vi "Mutate.vi"() -> ()   [LabVIEW 2014, in "VeriStand Steps Version Mutation.lvlib"]
uses:
  VeriStand Steps Version Mutation.lvlib
  Types/Version Build Information.ctl
  Types/Project Paths Cluster.ctl
  Types/dotNET Config File Paths Cluster.ctl
  <vilib>/Wiresmith Technology/LabVIEW CLI/CLI Class/CLI.lvclass
panel:
  out "error out":errorcluster
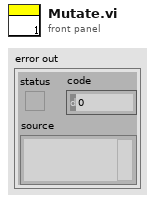
[diagram p1: front panel]
types:
  T1 = typedef "VeriStand Steps Version Mutation.lvlib/Version Build Information.ctl" = cluster{"VeriStand Version":string, "TestStand Version":string, "New VS Assembly Version":string, "New TS Assembly Version":string, "VeriStand Steps Version String":string, "Project Paths":T2, "New TS Interop Assembly Version":string, "New TS Utility Assembly Version":string, "New VS Assembly Version (GAC)":string, "dotNET .config File Paths":T3}
  T2 = typedef "VeriStand Steps Version Mutation.lvlib/Project Paths Cluster.ctl" = cluster{"MiscHelperVIs Project Path":string, "RTSequenceVIs Project Path":string, "Set Channels Project Path":string, "TS VS Logger Project Path":string, "VeriStand.exe Install Path":string, "NI_VeristandTypes.ini File Path":string, "Workspace Path":string, "VeristandSteps.csproj File Path":string, "Silent Veristand Project Path":string}
  T3 = typedef "VeriStand Steps Version Mutation.lvlib/dotNET Config File Paths Cluster.ctl" = cluster{"MiscHelperVIs Project .config File Path":path, "RT Sequence VIs Project .config File Path":path, "Set Channels Project .config File Path":path, "TS VS Logger Project .config File Path":path, "Silent Veristand Project .config File Path":path}
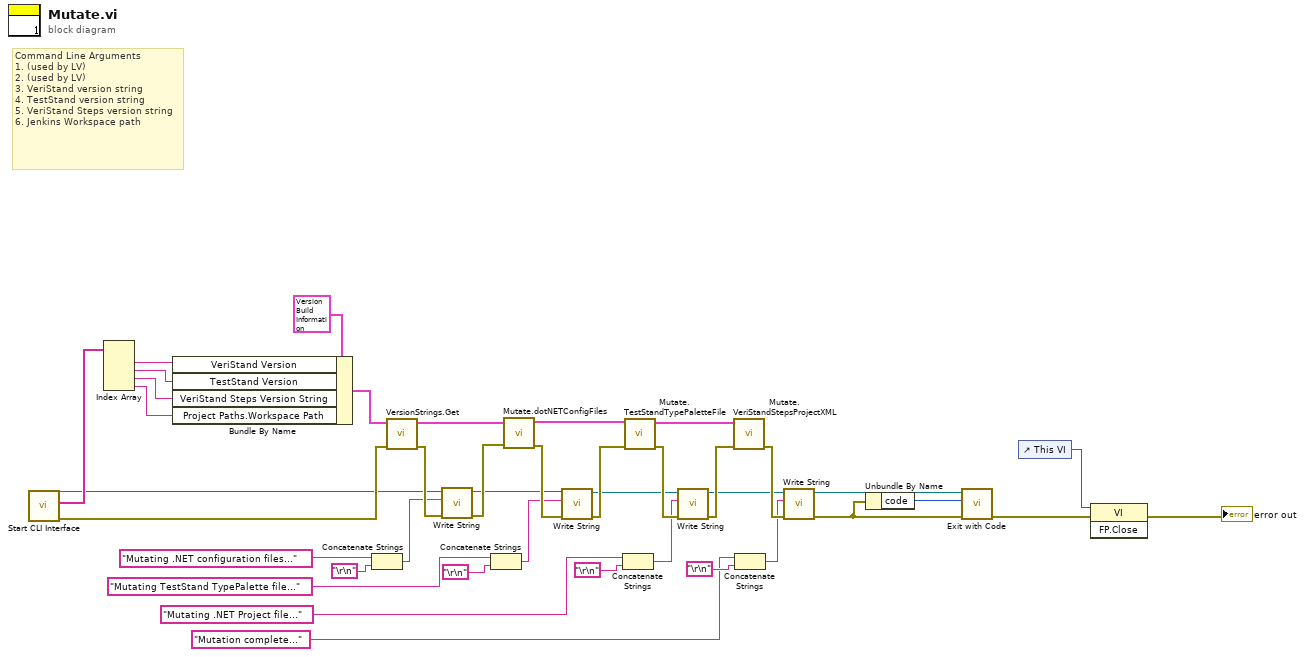
[diagram p0: block diagram]
diagram:
  # "Command Line Arguments\n1. (used by LV)\n2. (used by LV)\n3. VeriStand version string\n4. TestStand version string\n5. VeriStand Steps version string\n6. Jenkins Workspace path"
  n1 = call <vilib>:"Start CLI Interface.vi"() -> ("error out"=w32:errorcluster, "Custom Parameters"=w33:string[], "CLI out"=w25:refnum<class "CLI.lvclass">)  [unwired: 9 in]
  n2 = Index Array(array=w33) -> (element #1=w31:string, element #2=w30:string, element #3=w29:string, element #4=w28:string)  [unwired: 4 in]
  n3 = Bundle By Name(cluster=T1 {"VeriStand Version"="2013 SP1", "TestStand Version"="2013", "New VS Assembly Version"="2013.0.0.0", "New TS Assembly Version"="5.1.0.226", "VeriStand Steps Version String"="14.0.5.0", "Project Paths"={"MiscHelperVIs Project Path"="", "RTSequenceVIs Project Path"="", "Set Channels Project Path"="", "TS VS Logger Project Path"="", "VeriStand.exe Install Path"="", "NI_VeristandTypes.ini File Path"="", "Workspace Path"="", "VeristandSteps.csproj File Path"="", "Silent Veristand Project Path"=""}, "New TS Interop Assembly Version"="1.2.3.4", "New TS Utility Assembly Version"="5.6.7.8", "New VS Assembly Version (GAC)"="4.0.2016.0.9.9", "dotNET .config File Paths"={"MiscHelperVIs Project .config File Path"=path "C:/Users/Public/Documents/Git-Source/VeriStand-Custom-Steps-For-TestStand/Source/LabVIEW Code/Misc/MiscHelperVIs.lvproj.config", "RT Sequence VIs Project .config File Path"=path "C:/Users/Public/Documents/Git-Source/VeriStand-Custom-Steps-For-TestStand/Source/LabVIEW Code/RT Sequence/RTSequenceVIs.lvproj.config", "Set Channels Project .config File Path"=path "C:/Users/Public/Documents/Git-Source/VeriStand-Custom-Steps-For-TestStand/Source/LabVIEW Code/Set Channels/Set Channels.lvproj.config", "TS VS Logger Project .config File Path"=path "C:/Users/Public/Documents/Git-Source/VeriStand-Custom-Steps-For-TestStand/Source/LabVIEW Code/TS VS Logger/TS VS Logger.lvproj.config", "Silent Veristand Project .config File Path"=path "C:/Users/Public/Documents/Git-Source/VeriStand-Custom-Steps-For-TestStand/Source/LabVIEW Code/VeriStand Silent Start/SilentVS.lvproj.config"}} ("Version Build Information"), "VeriStand Version"=w31, "TestStand Version"=w30, "VeriStand Steps Version String"=w29, "Project Paths.Workspace Path"=w28) -> (w37:T1)
  n4 = Concatenate Strings("Mutating .NET configuration files..." ("Text to Write"), "\r\n") -> (w4:string)
  n5 = call "VersionStrings.Get.vi"("error in (no error)"=w32, "Version Build Information"=w37) -> ("error out"=w27:errorcluster, "Version Build Information out"=w36:T1)  [unwired: 8 in]
  n6 = call <vilib>:"Write String.vi"("error in (no error)"=w27, "Text to Write"=w4, "CLI in"=w25) -> ("error out"=w26:errorcluster, "CLI out"=w19:refnum<class "CLI.lvclass">)  [unwired: 7 in]
  n7 = Concatenate Strings("Mutating TestStand TypePalette file..." ("Text to Write"), "\r\n") -> (w3:string)
  n8 = call "Mutate.dotNETConfigFiles.vi"("error in (no error)"=w26, "Version Build Information"=w36) -> ("error out"=w24:errorcluster, "Version Build Information out"=w35:T1)  [unwired: 8 in]
  n9 = call <vilib>:"Write String.vi"("error in (no error)"=w24, "Text to Write"=w3, "CLI in"=w19) -> ("error out"=w23:errorcluster, "CLI out"=w18:refnum<class "CLI.lvclass">)  [unwired: 7 in]
  n10 = Concatenate Strings("Mutating .NET Project file..." ("Text to Write"), "\r\n") -> (w2:string)
  n11 = call "Mutate.TestStandTypePaletteFile.vi"("error in (no error)"=w23, "Version Build Information"=w35) -> ("error out"=w22:errorcluster, "Version Build Information out"=w34:T1)  [unwired: 8 in]
  n12 = call <vilib>:"Write String.vi"("error in (no error)"=w22, "Text to Write"=w2, "CLI in"=w18) -> ("error out"=w21:errorcluster, "CLI out"=w17:refnum<class "CLI.lvclass">)  [unwired: 7 in]
  n13 = call "Mutate.VeriStandStepsProjectXML.vi"("error in (no error)"=w21, "Version Build Info"=w34) -> ("error out"=w20:errorcluster)  [unwired: 8 in, 1 out]
  n14 = Concatenate Strings("Mutation complete..." ("Text to Write"), "\r\n") -> (w1:string)
  n15 = call <vilib>:"Write String.vi"("error in (no error)"=w20, "Text to Write"=w1, "CLI in"=w17) -> ("error out"=w13:errorcluster, "CLI out"=w16:refnum<class "CLI.lvclass">)  [unwired: 7 in]
  n16 = Unbundle By Name(w13) -> ("code"=w14:i32)
  n17 = call <vilib>:"Exit with Code.vi"("error in (no error)"=w13, "Exit Code (0)"=w14, "CLI in"=w16) -> ("error out"=w15:errorcluster)  [unwired: 8 in]
  n18 = control-ref of="This VI"() -> (w39:refnum<vi>)
  n19 = invoke class="VI" method="FP.Close"(reference=w39, error in=w15) -> (error out=→"error out":errorcluster)  [unwired: 1 in, 2 out]
